vi "Updated_File_Copy.vi"(2 "Target Path":path, 3 "Source Path":path) -> (0 "error in (no error)":errorcluster)   [LabVIEW 2010]
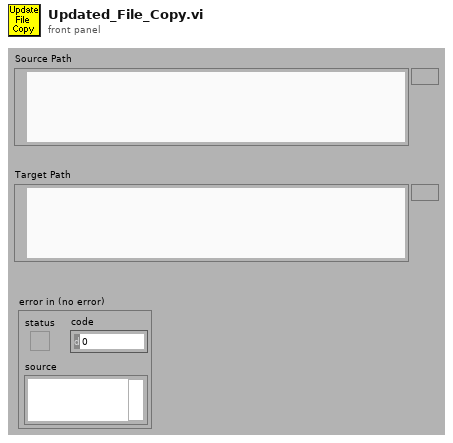
[diagram p1: front panel]
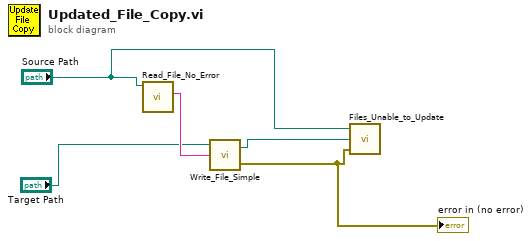
[diagram p0: block diagram]
diagram:
  n1 = call "Read_File_No_Error.vi"("Filename"="Source Path") -> ("string"=w5:string)  [unwired: 2 in, 7 out]
  n2 = call "Write_File_Simple.vi"("character string"=w5, "file path"="Target Path") -> ("error out"=w2:errorcluster, "file path Out"=w1:path)  [unwired: 1 in]
  "error in (no error)" <- w2
  n3 = call "Files_Unable_to_Update.vi"("error in (no error)"=w2, "Target Path"=w1, "Source Path"="Source Path") -> ()  [unwired: 1 out]
